vi "Setup Font.vi"(1 "Size":dbl=16.0, 2 "Font Path (System)":path, 3 "Font Name (First)":string) -> (0 "Font Settings out":refnum<class "Font Settings.lvclass">)   [LabVIEW 2020, in "Glyph Drawer.lvlib" / "Font Settings.lvclass"]
uses:
  Font Settings.lvclass
  Font Settings.lvclass/Font Settings.ctl
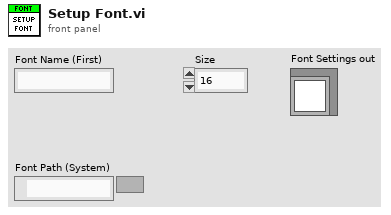
[diagram p1: front panel]
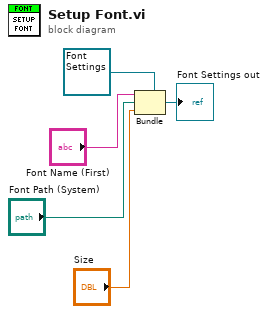
[diagram p0: block diagram]
diagram:
  n1 = Bundle(cluster=refnum<class "Font Settings.lvclass"> refnum ("Font Settings in"), "Font Name (First)", "Font Path (System)", "Size") -> (→"Font Settings out":refnum<class "Font Settings.lvclass">)
